vi "Read TSTRB Core.vi"(11 "niInstr AXI4-Stream Reader FXP64x4 v1 FPGA in":refnum<class "niInstr AXI4-Stream Reader FXP64x4 v1 FPGA.lvclass">) -> (2 "value":bool[](array[boolean]), 3 "niInstr AXI4-Stream Reader FXP64x4 v1 FPGA out":refnum<class "niInstr AXI4-Stream Reader FXP64x4 v1 FPGA.lvclass">)   [LabVIEW 2015, in "niInstr AXI4-Stream Reader FXP64x4 v1 FPGA.lvclass"]
uses:
  <instrlib>/_niInstr/CLIP Adapters/v1/FPGA/AXI4-Stream/Reader FXP64x4/niInstr AXI4-Stream Reader FXP64x4 v1 FPGA.lvclass
  <instrlib>/_niInstr/CLIP Adapters/v1/FPGA/AXI4-Stream/Reader FXP64x4/niInstr AXI4-Stream Reader FXP64x4 v1 FPGA.lvclass/niInstr AXI4-Stream Reader FXP64x4 v1 FPGA.ctl
  <instrlib>/_niInstr/Data Formatting/v1/FPGA/Private/Convert/U32 array to Boolean Array.vi
  <vilib>/rvi/eio/common/nirviEmuTemplateMethod_errors.vi
  <vilib>/eio/EIONode/EIONode.xnode
  <instrlib>/_niInstr/Data Formatting/v1/FPGA/niInstr Data Formatting v1 FPGA.lvlib
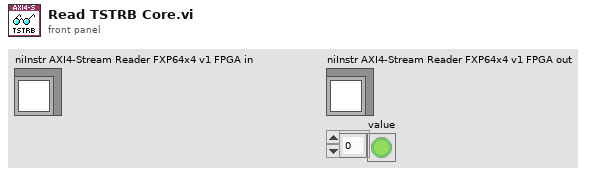
[diagram p1: front panel]
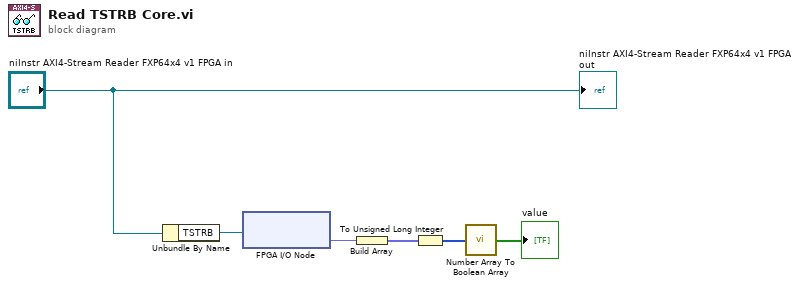
[diagram p0: block diagram]
diagram:
  n1 = Unbundle By Name("niInstr AXI4-Stream Reader FXP64x4 v1 FPGA in") -> ("TSTRB"=w5:refnum<k21>)
  n2 = xnode "FPGA I/O Node"("FPGA I/O In"=w5) -> ("I/O Item"=w6:fxp<+,32,32>)  [unwired: 1 out]
  n3 = Build Array(w6) -> (w2:fxp<+,32,32>[])
  n4 = To Unsigned Long Integer(number=w2) -> (unsigned 32bit integer=w1:u32[])
  n5 = call-poly <instrlib>:"Number Array To Boolean Array.vi"("data in"=w1) -> ("data out"=→"value":bool[])  [unwired: 14 in]
  "niInstr AXI4-Stream Reader FXP64x4 v1 FPGA out" <- "niInstr AXI4-Stream Reader FXP64x4 v1 FPGA in"
